vi "Get-FP-All-Ctrl-Ref.vi"(8 "error in (no error)":errorcluster, 11 "VI Refnum":refnum<vi>) -> (0 "error out":errorcluster, 3 "Quick-GUI-Update out":refnum<class "Quick-GUI-Update.lvclass">)   [LabVIEW 2020, in "Easy GUI Operation.lvlib" / "Quick-GUI-Update.lvclass"]
uses:
  Quick-GUI-Update.lvclass
  Quick-GUI-Update.lvclass/Quick-GUI-Update.ctl
  <vilib>/Utility/miscctls.llb/LVMapReplaceAction.ctl
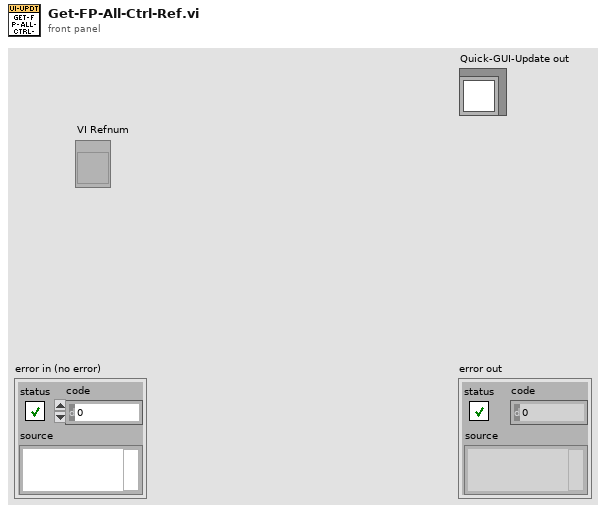
[diagram p1: front panel]
types:
  T1 = typedef "LVMapReplaceAction.ctl" = enum32{"Modify Entry only if found", "Add or Modify Entry", "Delete Entry"}
  T2 = cluster{"Ctrl-Ref":refnum<vi>, "Ctrl Index":i32, "Class-Name":string, "Class ID":u32}
  T3 = map{string, set{cluster{"Ctrl-Ref":refnum<vi>, "Ctrl Index":i32, "Class-Name":string, "Class ID":u32}}}
  T4 = set{cluster{"Ctrl-Ref":refnum<vi>, "Ctrl Index":i32, "Class-Name":string, "Class ID":u32}}
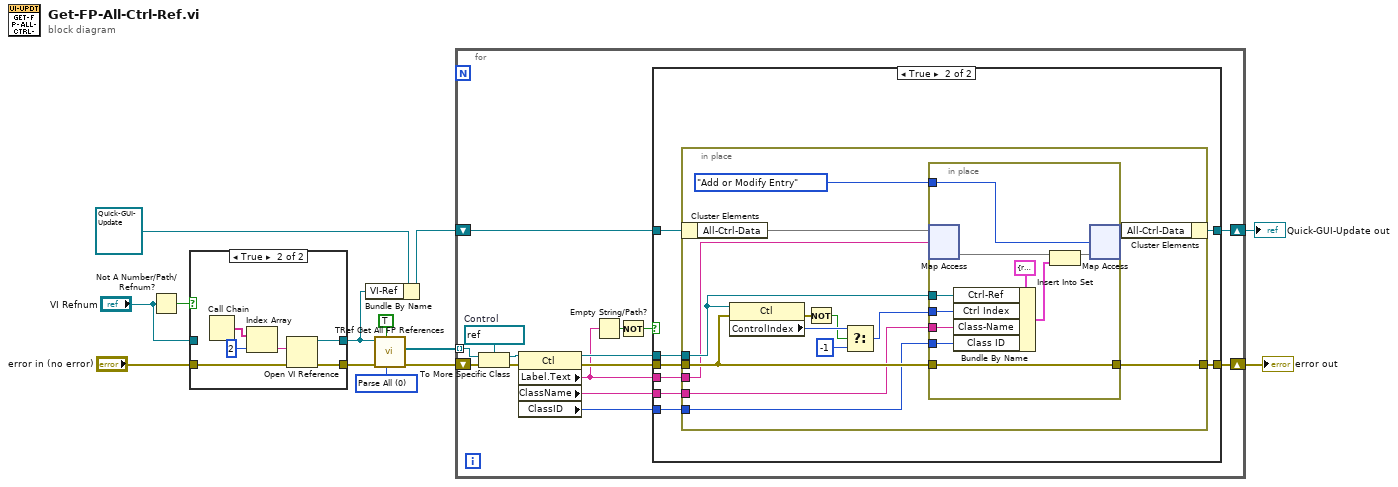
[diagram p0: block diagram]
diagram:
  w5 = u16 0 items=["Parse All", "Parse Tabs Only"] ("Parsing Rule")
  n1 = Not A Number/Path/Refnum?(number/path/refnum="VI Refnum") -> (NaN/Path/Refnum?=w8:bool)
  n2 = case shown="True" w8 {
    tunnel: "VI Refnum" -> [w15 _]
    tunnel: [w15 w16] -> w4
    tunnel: "error in (no error)" -> [w14 w18]
    tunnel: [w14 w17] -> w7
    frame False {
    }
    frame True {
      n3 = Call Chain() -> (call chain=w21:string[])
      n4 = Index Array(array=w21, index=2 ("Index")) -> (element=w20:string)
      n5 = Open VI Reference(vi path=w20, error in (no error)=w18) -> (vi reference=w16:refnum<vi>, error out=w17:errorcluster)  [unwired: 4 in]
    }
  }
  n6 = Bundle By Name(cluster=refnum<class "Quick-GUI-Update.lvclass"> refnum ("Quick-GUI-Update in"), "VI-Ref"=w4) -> (w3:refnum<class "Quick-GUI-Update.lvclass">)
  n7 = call <vilib>:"TRef Get All FP References.vi"("Parsing Rule"=w5, "Ignore Decorations?"=TRUE, "error in (no error)"=w7, "VI Refnum"=w4) -> ("error out"=w2:errorcluster, "All FP Objects"=w1:refnum<vi>[])  [unwired: 3 in, 3 out]
  n8 = for {
    tunnel: w1 -> [w27] mode=indexing
    shift-right: [w25] -> w12
    shift-left: w2 -> [w35]
    shift-right: [w26] -> w10
    shift-left: w3 -> [w34]
    w36 = refnum<vi> refnum  # Control
    n9 = To More Specific Class(target class=w36, reference=w27, error in=w35) -> (specific class reference=w33:refnum<vi>, error out=w31:errorcluster)
    n10 = property class="Ctl"(reference=w33, error in=w31) -> (reference out=w32:refnum<vi>, error out=w30:errorcluster, "Label.Text"=w23:string, "ClassName"=w24:string, "ClassID"=w22:u32)
    n11 = Empty String/Path?(string/path=w23) -> (empty?=w29:bool)
    n12 = Not(x=w29) -> (.not. x?=w28:bool)
    n13 = case shown="True" w28 {
      tunnel: w34 -> [w38 w46]
      tunnel: w32 -> [_ w45]
      tunnel: w30 -> [w37 w44]
      tunnel: w24 -> [_ w42]
      tunnel: w23 -> [_ w43]
      tunnel: [w38 w41] -> w26
      tunnel: [w37 w40] -> w25
      tunnel: w22 -> [_ w39]
      frame False {
      }
      frame True {
        n14 = in-place {
          in-place-border: [w52] -> w40
          in-place-border: w45 -> [w55]
          in-place-border: w44 -> [w51]
          in-place-border: w43 -> [w49]
          in-place-border: w42 -> [w48]
          in-place-border: w39 -> [w47]
          n15 = in-place-cluster #1(w46) -> ("All-Ctrl-Data"=w56:T3)
          n16 = property class="Ctl"(reference=w55, error in=w51) -> (error out=w60:errorcluster, "ControlIndex"=w59:i32)  [unwired: 1 out]
          n17 = Not(x=w60) -> (.not. x?=w57:bool)
          n18 = Select(t=w59, s=w57, f=-1) -> (s? t:f=w54:i32)
          n19 = in-place {
            in-place-border: w55 -> [w70]
            in-place-border: w54 -> [w69]
            in-place-border: [w68] -> w52
            in-place-border: w51 -> [w68]
            in-place-border: LVMapReplaceAction."Add or Modify Entry" ("action") -> [w66]
            in-place-border: w48 -> [w67]
            in-place-border: w47 -> [w61]
            n20 = in-place-map #2(w56, w49) -> (w63:T4)  [unwired: 1 in, 1 out]
            n21 = Bundle By Name(cluster=T2 {"Ctrl-Ref"=refnum, "Ctrl Index"=0, "Class-Name"="", "Class ID"=0} ("element"), "Ctrl-Ref"=w70, "Ctrl Index"=w69, "Class-Name"=w67, "Class ID"=w61) -> (w64:T2)
            n22 = Insert Into Set(10:w64, 11:w63) -> (3:w62:T4)  [unwired: 1 out]
            n23 = in-place-map #2(w62, w66) -> (w53:T3)  [unwired: 2 out]
          }
          n24 = in-place-cluster #1("All-Ctrl-Data"=w53) -> (w41:refnum<class "Quick-GUI-Update.lvclass">)
        }
      }
    }
  }
  "error out" <- w12
  "Quick-GUI-Update out" <- w10
